vi "Test Lists Updated.vi"(11 "Result Model Result Recording Test in":refnum<class "Result Model Result Recording Test.lvclass">) -> (0 "error out":errorcluster, 3 "Result Model Result Recording Test out":refnum<class "Result Model Result Recording Test.lvclass">)   [LabVIEW 2020, in "Result Model Result Recording Test.lvclass"]
uses:
  Result Model Result Recording Test.lvclass
  C:/Program Files (x86)/National Instruments/LabVIEW 2020/vi.lib/Astemes/LUnit/Test Case.lvclass
  <vilib>/Astemes/LUnit/Test Case.lvclass/Test Case.ctl
  ae2c71b8-32bb-49d1-8500-0119bfec74ff.vi
  <vilib>/Astemes/LUnit/Core/LUnit Test Case/Private/Append Pass Result.vi
  <vilib>/Astemes/LUnit/Core/LUnit Test Case/Private/Append Fail Result.vi
  ae2c71b8-32bb-49d1-8500-0119bfec74ff.vi/9c5d11cd-9439-4240-a1ee-d9baace9c924.vi
  <vilib>/Astemes/LUnit/Core/LUnit Test Case/Private/Run In UI.vi
  <vilib>/Utility/error.llb/Clear Errors.vi
  source/User Interface/Result Model by Reference/Result Model by Reference.lvclass
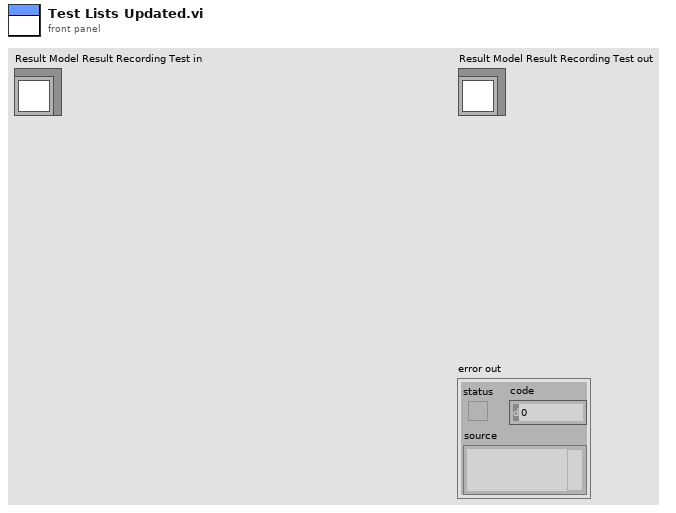
[diagram p1: front panel]
types:
  T1 = cluster{"Left Cell String":string, "Child Text":string[], "Child Tag":string, "Item Indent":i32, "Child Only?":bool, "Glyph Index":i32}[]
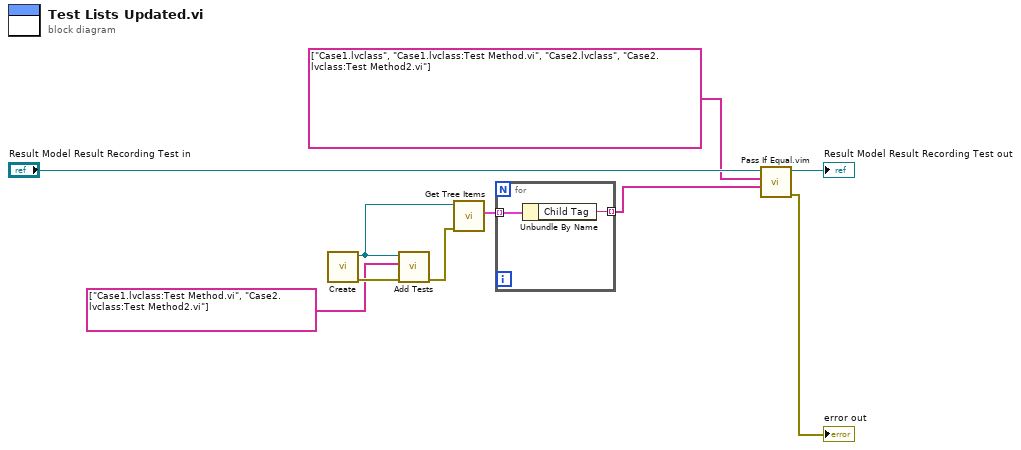
[diagram p0: block diagram]
diagram:
  n1 = call "Create.vi"() -> ("error out"=w3:errorcluster, "Result Model out"=w10:refnum<class "Result Model by Reference.lvclass">)  [unwired: 10 in]
  n2 = call "Add Tests.vi"("error in (no error)"=w3, "Tests"=string[] ["Case1.lvclass:Test Method.vi", "Case2.lvclass:Test Method2.vi"], "Result Model by Reference In"=w10) -> ("error out"=w1:errorcluster)  [unwired: 8 in]
  n3 = call "Get Tree Items.vi"("error in (no error)"=w1, "Result Model by Reference In"=w10) -> ("Tree Items"=w9:T1)  [unwired: 8 in, 1 out]
  n4 = for {
    tunnel: w9 -> [w12] mode=indexing
    tunnel: [w11] -> w5 mode=indexing
    n5 = Unbundle By Name(w12) -> ("Child Tag"=w11:string)
  }
  n6 = call "Pass If Equal.vim"("Actual"=w5, "Expected"=string[] ["Case1.lvclass", "Case1.lvclass:Test Method.vi", "Case2.lvclass", "Case2.lvclass:Test Method2.vi"], "LUnit Test Case In"="Result Model Result Recording Test in") -> ("error out"=→"error out":errorcluster, "LUnit Test Case Out"=→"Result Model Result Recording Test out":refnum<class "Result Model Result Recording Test.lvclass">)  [unwired: 7 in]
